vi "UpdateAllDeviceList.vi"(0 "nTimeOut":u32, 1 "error in (no error)":errorcluster) -> (2 "punNumDevices":i32, 3 "GX_STATUS":i32, 4 "error out":errorcluster)   [LabVIEW 2016, in "GxLVLib.lvlib"]
uses:
  GxLVLib.lvlib
  GxIAPI.dll
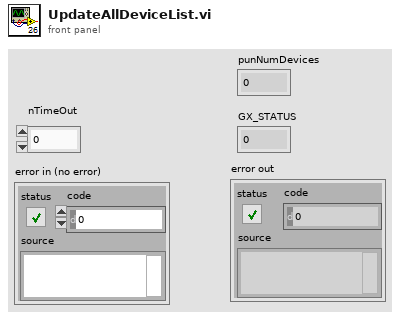
[diagram p1: front panel]
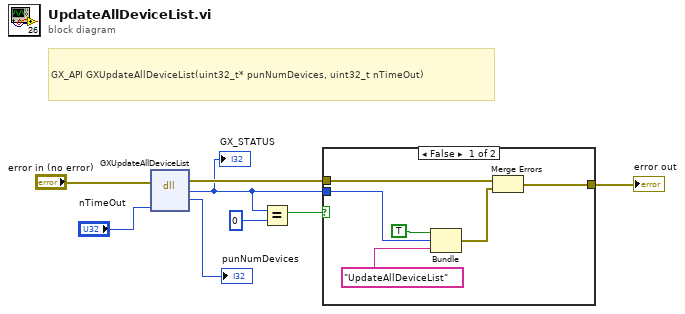
[diagram p0: block diagram]
diagram:
  # "GX_API GXUpdateAllDeviceList(uint32_t* punNumDevices, uint32_t nTimeOut)"
  n1 = dll-call lib="GxIAPI.dll" fn="GXUpdateAllDeviceList"(error in="error in (no error)", "nTimeOut"="nTimeOut") -> (error out=w5:errorcluster, "GX_STATUS"=w1:i32, "punNumDevices"=→"punNumDevices":u32)  [unwired: 4 in, 1 out]
  "GX_STATUS" <- w1
  n2 = Equal?(x=w1, y=0) -> (x = y?=w3:bool)
  n3 = case shown="False" w3 {
    tunnel: w5 -> [w14 w15]
    tunnel: [w13 w15] -> w2
    tunnel: w1 -> [w10 _]
    frame False {
      n4 = Bundle(TRUE, "GX_STATUS"=w10, "UpdateAllDeviceList") -> (w11:cluster{bool, "GX_STATUS":i32, string})  [unwired: 1 in]
      n5 = Merge Errors(w14, w11) -> (w13:errorcluster)
    }
    frame True {
    }
  }
  "error out" <- w2
